vi "PH_SHS_Analysis_Calibrator.ProcState.vi"(0 "i ref in":refnum<vi>, 2 "state timeout":i32=-1, 4 "state":string, 5 "error in (no error)":errorcluster) -> (14 "i ref out":refnum<vi>, 18 "next state":string, 19 "error out":errorcluster)   [LabVIEW 2014, in "PH_SHS_Analysis_Calibrator.lvlib"]
doc: "This VI represents part of the internal state machine of the object. All methods that are needed to implement the required functionality of the state machine will be called from THIS VI. Add your code here."
uses:
  PH_SHS_Analysis_Calibrator.lvlib
  CSCore/CSSystem/CoreDefs/CoreDefs.error_type.ctl
  CSCore/CSSystem/CoreLib/CoreLib.lvlib
  CSCore/BaseSM/BaseSM.lvlib
  CSCore/BaseProcess/BaseProcess.lvlib
  CSCore/CSSystem/CSSystemLib/CSSystemLib.lvlib
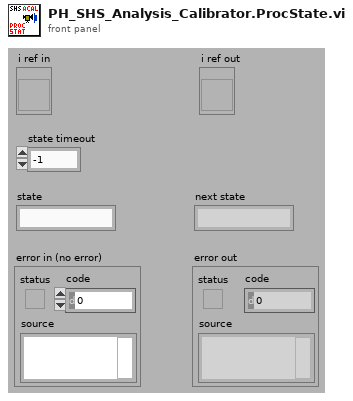
[diagram p1: front panel]
types:
  T1 = enum16{"simple", "synchronous", "asynchronous", "notification"}
  T2 = typedef "CoreDefs.error_type.ctl" = enum16{"no error", "can't load process", "can't unload process", "process does not exist", "can't install process", "can't remove process", "unknown function", "time out", "can't execute function", "duplicate queue name", "super not found", "caller queue invalid", "can't ping process", "unknown error", "VISA Error", "VISA timeout", "GPIB timeout", "GPIB error", "communication error", "data type mismatch", "can't read data from OPC server", "can't write data to OPC server", "OET error", "function not implemented", "process already exists", "invalid Shared Variable name", "error writing Shared Variable", "error reading Shared Variable", "invalid client name", "corrupt database", "unknown class", "call not authorized", "parameter out of range", "OET timeout: can't get data to modify", "invalid queue name", "requested operation incompatible with current state", "event undefined", "event disabled", "state undefined", "caller is not a friend", "EventBuilder: bad eventID", "EventBuilder: no DAQ devices", "a thread must not stop itself", "UNUSED ELEMENT4", "DiscArchiver: eventData incomplete", "DiscArchiver: eventData does not belong to run", "DiscArchiver: can't open file", "DiscArchiver: can't write to file", "DiscArchiver: available disc space low", "can't acquire semaphore", "error reading data from database", "notifier object is not existing", "can't register process", "can't unregister process", "illegal event type", "object disabled", "object already exists", "can't change state", "Instrument not found", "no connection to remote node", "invalid reference", "N/A", "UNUSED ELEMENT 1", "element not found", "illegal TCP/IP connection detected", "object does not exist", "invalid access ID", "unknown CS system", "invalid privilige", "unsupported data type", "unsupported server type", "IO server already exists", "Shared Variable already exists"}
  T3 = typedef "PH_SHS_Analysis_Calibrator.lvlib/PH_SHS_Analysis_Calibrator.i attribute.ctl" = cluster{"GUI Refs":cluster{"Available Cams":refnum<vi>, "OK":refnum<vi>, "Skip":refnum<vi>, "Repeat":refnum<vi>, "Cancel":refnum<vi>, "Dialog":refnum<vi>, "Enough Images?":refnum<vi>}, "Cam instances":string[], "Status":cluster{"#":i32, "Data calculated":bool, "Wanted #":i32}, "IMAQ Image Array":T4[], "Pixel Size [µm]":dbl, "MLA Pitch [µm]":dbl, "Method":enum16{"automatic", "manual"}, "Enough Images?":bool, "SHS Reference Result":T5, "Calculation Error":errorcluster}
  T4 = typedef "IMAQ Image.ctl" = refnum<image>
  T5 = typedef "SHS_Common.lvlib/SHSReference.ctl" = cluster{"Reference":T6[][], "Lens Array Pitch [px]":dbl}
  T6 = typedef "SHS_Common.lvlib/ReferencePoint.ctl" = cluster{"Rect":T7, "Point":T8}
  T7 = typedef "SHS_Common.lvlib/Rectangle.ctl" = cluster{"Left":i32, "Top":i32, "Right":i32, "Bottom":i32}
  T8 = typedef "SHS_Common.lvlib/Point.ctl" = cluster{"x":dbl, "y":dbl, "valid?":bool, "weight":dbl}
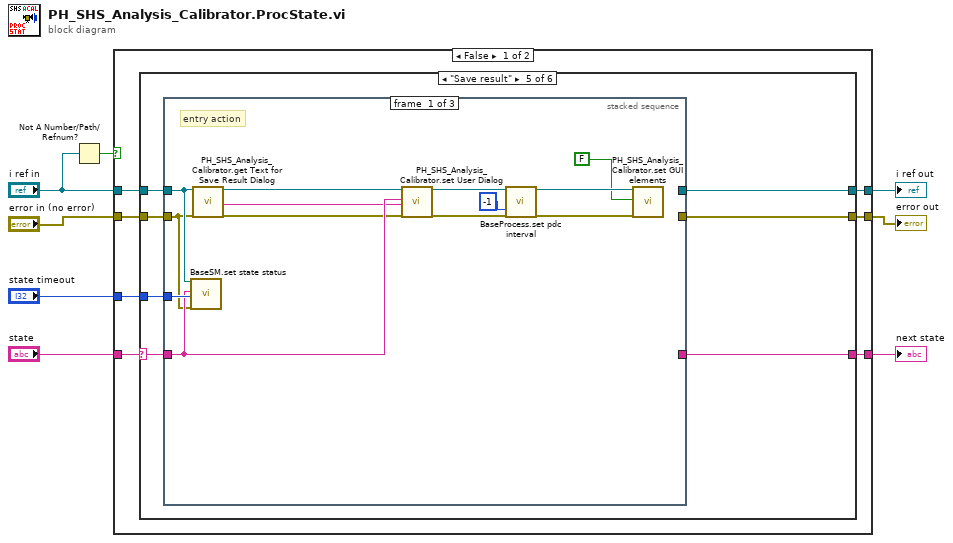
[diagram p0: block diagram]
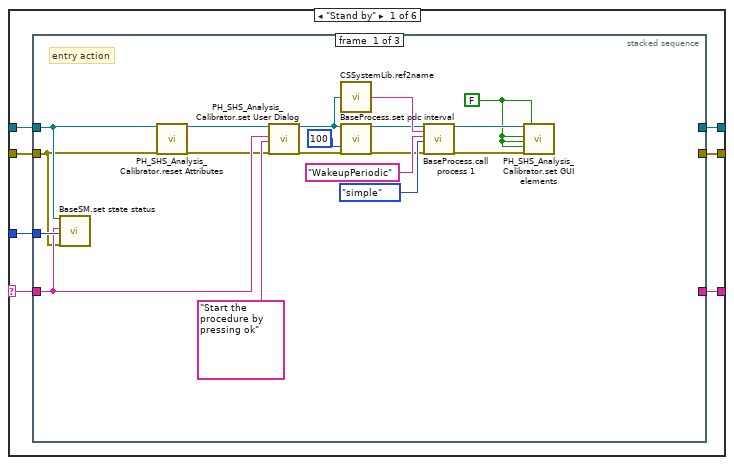
[diagram p2: hidden frame]
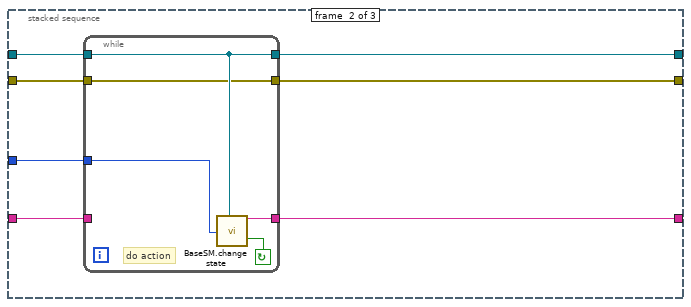
[diagram p3: hidden frame]
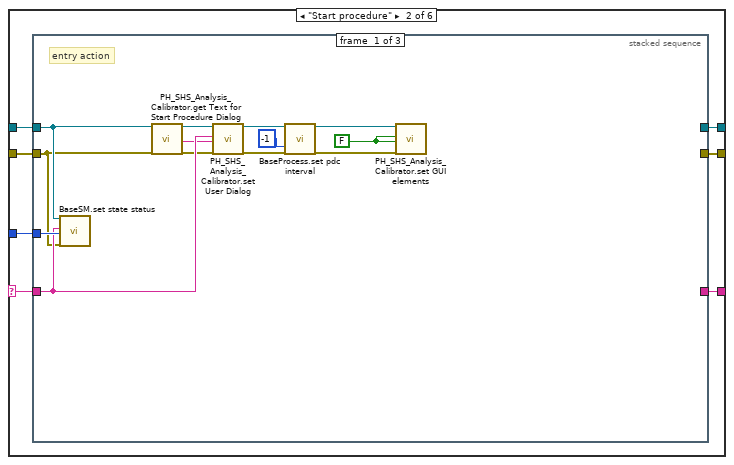
[diagram p5: hidden frame]
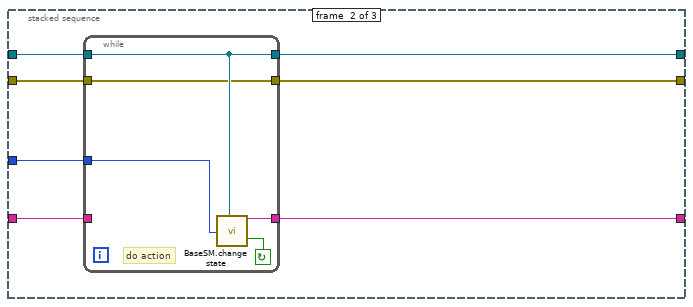
[diagram p6: hidden frame]
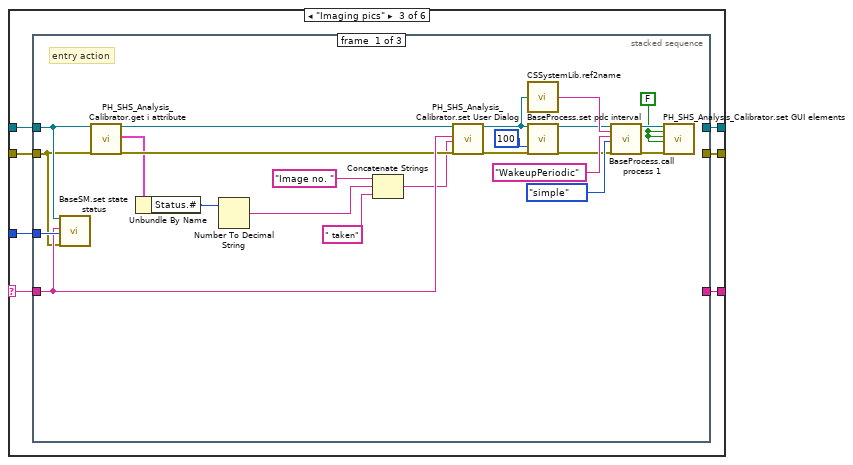
[diagram p8: hidden frame]
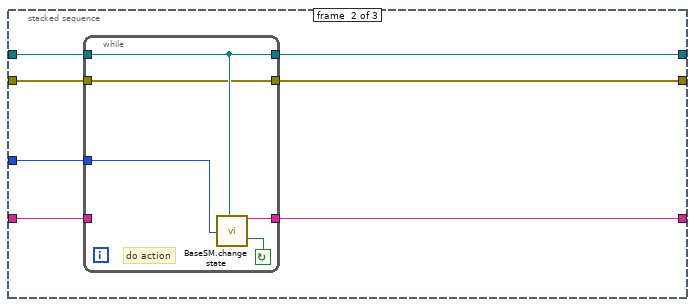
[diagram p9: hidden frame]
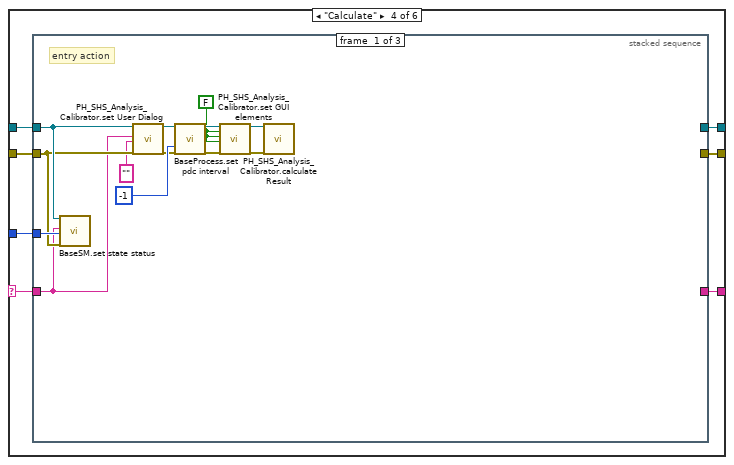
[diagram p11: hidden frame]
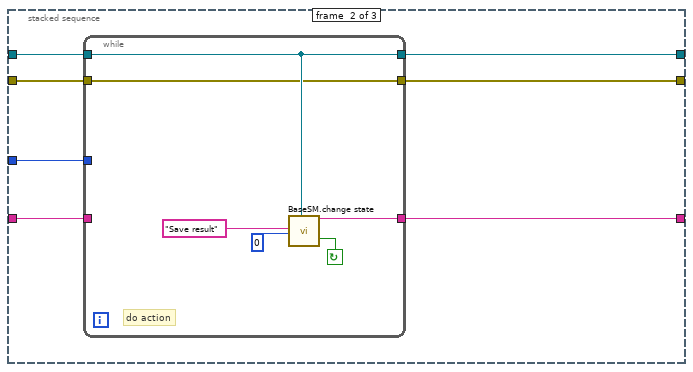
[diagram p12: hidden frame]
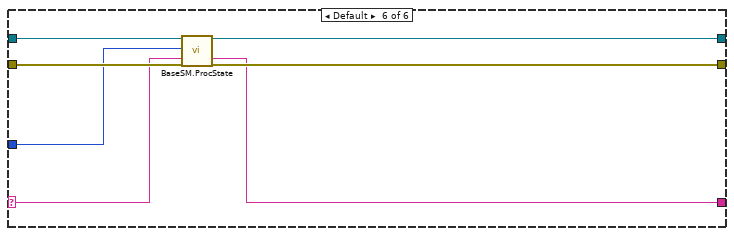
[diagram p16: hidden frame]
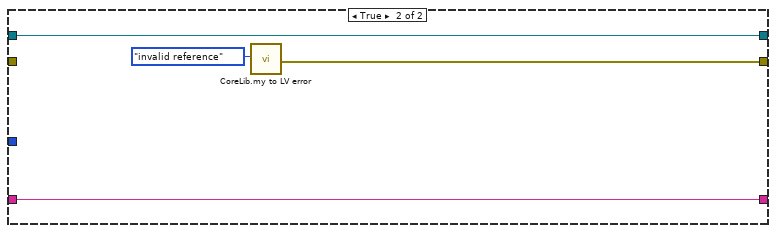
[diagram p17: hidden frame]
diagram:
  n1 = Not A Number/Path/Refnum?(number/path/refnum="i ref in") -> (NaN/Path/Refnum?=w2:bool)
  n2 = case shown="False" w2 {
    tunnel: "i ref in" -> [w15 w202]
    tunnel: [w14 w202] -> w8
    tunnel: "state" -> [w13 w199]
    tunnel: [w12 w199] -> w6
    tunnel: "state timeout" -> [w11 _]
    tunnel: "error in (no error)" -> [w10 _]
    tunnel: [w9 w200] -> w3
    frame False {
      n3 = case shown="\"Save result\"" w13 {
        selector: w13 -> [w22 w59 w91 w133 w166 w193]
        tunnel: w15 -> [w20 w57 w89 w131 w164 w198]
        tunnel: [w19 w56 w88 w130 w163 w197] -> w14
        tunnel: [w21 w58 w90 w132 w165 w192] -> w12
        tunnel: w11 -> [w18 w55 w87 w129 w162 w194]
        tunnel: w10 -> [w17 w54 w86 w128 w161 w196]
        tunnel: [w16 w53 w85 w127 w160 w195] -> w9
        frame "Stand by" {
          n4 = stacked-sequence {
            tunnel: w22 -> [w39 w47 _]
            tunnel: [_ w46 _] -> w21
            tunnel: w20 -> [w26 w44 _]
            tunnel: [_ w43 _] -> w19
            tunnel: w18 -> [w40 w45 _]
            tunnel: w17 -> [w24 w41 _]
            tunnel: [_ w42 _] -> w16
            frame #0 {
              w27 = FALSE ("Cams disabled (true)")
              # "entry action"
              n5 = call "BaseSM.set state status.vi"("i ref in"=w26, "stateStatus"=w39, "ms timeout (10000)"=w40, "error in (no error)"=w24) -> ()  [unwired: 13 in, 3 out]
              n6 = call "PH_SHS_Analysis_Calibrator.reset Attributes.vi"("i ref in"=w26, "error in (no error)"=w24) -> ("i ref out"=w25:refnum<vi>, "error out"=w23:errorcluster)  [unwired: 16 in]
              n7 = call "PH_SHS_Analysis_Calibrator.set User Dialog.vi"("i ref in"=w25, "State"=w39, "Text"="Start the procedure by pressing ok", "error in (no error)"=w23) -> ("i ref out"=w31:refnum<vi>, "error out"=w33:errorcluster)  [unwired: 14 in]
              n8 = call "CSSystemLib.ref2name.vi"("obj refnum"=w31) -> ("name"=w37:string)
              n9 = call "BaseProcess.set pdc interval.vi"("i ref in"=w31, "PeriodicInterval [ms]"=100 ("PeriodicInterval"), "error in (no error)"=w33) -> ("i ref out"=w32:refnum<vi>, "error out"=w34:errorcluster)  [unwired: 14 in, 1 out]
              n10 = call "BaseProcess.call process 1.vi"("i ref in"=w32, "Object"=w37, "Selector"="WakeupPeriodic", "CallType"=T1."simple", "error in (no error)"=w34) -> ("i ref out"=w29:refnum<vi>, "error out"=w28:errorcluster)  [unwired: 12 in, 1 out]
              n11 = call "PH_SHS_Analysis_Calibrator.set GUI elements.vi"("i ref in"=w29, "skip visible (true)"=w27, "Repeat visible (true)"=w27, "Cancel visible (true)"=w27, "error in (no error)"=w28, "Cams disabled (true)"=w27) -> ()  [unwired: 12 in, 2 out]
            }
            frame #1 {
              n12 = while {
                tunnel: w45 -> [w50]
                tunnel: [w52] -> w46
                tunnel: w47 -> [_]
                tunnel: w44 -> [w49]
                tunnel: [w49] -> w43
                tunnel: [w48] -> w42
                tunnel: w41 -> [w48]
                stop <- w51 continue-if-true
                # "do action"
                n13 = call "BaseSM.change state.vi"("wait time [ms]"=w50, "i ref in"=w49) -> ("next state"=w52:string, "continue loop"=w51:bool)  [unwired: 14 in, 2 out]
              }
            }
            frame #2 {
              # "exit action"
            }
          }
        }
        frame "Start procedure" {
          n14 = stacked-sequence {
            tunnel: w59 -> [w71 w79 _]
            tunnel: [_ w78 _] -> w58
            tunnel: w57 -> [w65 w76 _]
            tunnel: [_ w75 _] -> w56
            tunnel: w55 -> [w72 w77 _]
            tunnel: w54 -> [w63 w73 _]
            tunnel: [_ w74 _] -> w53
            frame #0 {
              w60 = FALSE ("Repeat visible (true)")
              # "entry action"
              n15 = call "BaseSM.set state status.vi"("i ref in"=w65, "stateStatus"=w71, "ms timeout (10000)"=w72, "error in (no error)"=w63) -> ()  [unwired: 13 in, 3 out]
              n16 = call "PH_SHS_Analysis_Calibrator.get Text for Start Procedure Dialog.vi"("i ref in"=w65, "error in (no error)"=w63) -> ("i ref out"=w64:refnum<vi>, "Dialog Start Procedure"=w61:string, "error out"=w62:errorcluster)  [unwired: 15 in]
              n17 = call "PH_SHS_Analysis_Calibrator.set User Dialog.vi"("i ref in"=w64, "State"=w71, "Text"=w61, "error in (no error)"=w62) -> ("i ref out"=w68:refnum<vi>, "error out"=w69:errorcluster)  [unwired: 14 in]
              n18 = call "BaseProcess.set pdc interval.vi"("i ref in"=w68, "PeriodicInterval [ms]"=-1 ("PeriodicInterval"), "error in (no error)"=w69) -> ("i ref out"=w67:refnum<vi>, "error out"=w66:errorcluster)  [unwired: 14 in, 1 out]
              n19 = call "PH_SHS_Analysis_Calibrator.set GUI elements.vi"("i ref in"=w67, "skip visible (true)"=w60, "Repeat visible (true)"=w60, "error in (no error)"=w66) -> ()  [unwired: 14 in, 2 out]
            }
            frame #1 {
              n20 = while {
                tunnel: w77 -> [w82]
                tunnel: [w84] -> w78
                tunnel: w79 -> [_]
                tunnel: w76 -> [w81]
                tunnel: [w81] -> w75
                tunnel: [w80] -> w74
                tunnel: w73 -> [w80]
                stop <- w83 continue-if-true
                # "do action"
                n21 = call "BaseSM.change state.vi"("wait time [ms]"=w82, "i ref in"=w81) -> ("next state"=w84:string, "continue loop"=w83:bool)  [unwired: 14 in, 2 out]
              }
            }
            frame #2 {
              # "exit action"
            }
          }
        }
        frame "Imaging pics" {
          n22 = stacked-sequence {
            tunnel: w91 -> [w113 w121 _]
            tunnel: [_ w120 _] -> w90
            tunnel: w89 -> [w112 w118 _]
            tunnel: [_ w117 _] -> w88
            tunnel: w87 -> [w114 w119 _]
            tunnel: w86 -> [w110 w115 _]
            tunnel: [_ w116 _] -> w85
            frame #0 {
              w92 = FALSE ("ok visible (true)")
              # "entry action"
              n23 = call "BaseSM.set state status.vi"("i ref in"=w112, "stateStatus"=w113, "ms timeout (10000)"=w114, "error in (no error)"=w110) -> ()  [unwired: 13 in, 3 out]
              n24 = call "PH_SHS_Analysis_Calibrator.get i attribute.vi"("i ref in"=w112, "error in (no error)"=w110) -> ("i ref out"=w111:refnum<vi>, "i attribute"=w108:T3, "error out"=w109:errorcluster)  [unwired: 15 in]
              n25 = Unbundle By Name(w108) -> ("Status.#"=w107:i32)
              n26 = Number To Decimal String(number=w107) -> (decimal integer string=w105:string)  [unwired: 1 in]
              n27 = Concatenate Strings("Image no. " ("string"), w105, " taken" ("string")) -> (w103:string)
              n28 = call "PH_SHS_Analysis_Calibrator.set User Dialog.vi"("i ref in"=w111, "State"=w113, "Text"=w103, "error in (no error)"=w109) -> ("i ref out"=w96:refnum<vi>, "error out"=w95:errorcluster)  [unwired: 14 in]
              n29 = call "CSSystemLib.ref2name.vi"("obj refnum"=w96) -> ("name"=w101:string)
              n30 = call "BaseProcess.set pdc interval.vi"("i ref in"=w96, "PeriodicInterval [ms]"=100 ("PeriodicInterval"), "error in (no error)"=w95) -> ("i ref out"=w97:refnum<vi>, "error out"=w98:errorcluster)  [unwired: 14 in, 1 out]
              n31 = call "BaseProcess.call process 1.vi"("i ref in"=w97, "Object"=w101, "Selector"="WakeupPeriodic", "CallType"=T1."simple", "error in (no error)"=w98) -> ("i ref out"=w94:refnum<vi>, "error out"=w93:errorcluster)  [unwired: 12 in, 1 out]
              n32 = call "PH_SHS_Analysis_Calibrator.set GUI elements.vi"("i ref in"=w94, "ok visible (true)"=w92, "skip visible (true)"=w92, "Repeat visible (true)"=w92, "error in (no error)"=w93) -> ()  [unwired: 13 in, 2 out]
            }
            frame #1 {
              n33 = while {
                tunnel: w119 -> [w124]
                tunnel: [w126] -> w120
                tunnel: w121 -> [_]
                tunnel: w118 -> [w123]
                tunnel: [w123] -> w117
                tunnel: [w122] -> w116
                tunnel: w115 -> [w122]
                stop <- w125 continue-if-true
                # "do action"
                n34 = call "BaseSM.change state.vi"("wait time [ms]"=w124, "i ref in"=w123) -> ("next state"=w126:string, "continue loop"=w125:bool)  [unwired: 14 in, 2 out]
              }
            }
            frame #2 {
              # "exit action"
            }
          }
        }
        frame "Calculate" {
          n35 = stacked-sequence {
            tunnel: w133 -> [w143 w153 _]
            tunnel: [_ w152 _] -> w132
            tunnel: w131 -> [w145 w150 _]
            tunnel: [_ w149 _] -> w130
            tunnel: w129 -> [w146 w151 _]
            tunnel: w128 -> [w144 w147 _]
            tunnel: [_ w148 _] -> w127
            frame #0 {
              w136 = FALSE ("ok visible (true)")
              # "entry action"
              n36 = call "BaseSM.set state status.vi"("i ref in"=w145, "stateStatus"=w143, "ms timeout (10000)"=w146, "error in (no error)"=w144) -> ()  [unwired: 13 in, 3 out]
              n37 = call "PH_SHS_Analysis_Calibrator.set User Dialog.vi"("i ref in"=w145, "State"=w143, "Text"="", "error in (no error)"=w144) -> ("i ref out"=w140:refnum<vi>, "error out"=w141:errorcluster)  [unwired: 14 in]
              n38 = call "BaseProcess.set pdc interval.vi"("i ref in"=w140, "PeriodicInterval [ms]"=-1 ("PeriodicInterval"), "error in (no error)"=w141) -> ("i ref out"=w139:refnum<vi>, "error out"=w138:errorcluster)  [unwired: 14 in, 1 out]
              n39 = call "PH_SHS_Analysis_Calibrator.set GUI elements.vi"("i ref in"=w139, "ok visible (true)"=w136, "skip visible (true)"=w136, "Repeat visible (true)"=w136, "error in (no error)"=w138) -> ("i ref out"=w135:refnum<vi>, "error out"=w134:errorcluster)  [unwired: 13 in]
              n40 = call "PH_SHS_Analysis_Calibrator.calculate Result.vi"("i ref in"=w135, "error in"=w134) -> ()  [unwired: 16 in, 2 out]
            }
            frame #1 {
              n41 = while {
                tunnel: w151 -> [_]
                tunnel: [w159] -> w152
                tunnel: w153 -> [_]
                tunnel: w150 -> [w157]
                tunnel: [w157] -> w149
                tunnel: [w156] -> w148
                tunnel: w147 -> [w156]
                stop <- w158 continue-if-true
                # "do action"
                n42 = call "BaseSM.change state.vi"("default state"="Save result", "wait time [ms]"=0, "i ref in"=w157) -> ("next state"=w159:string, "continue loop"=w158:bool)  [unwired: 13 in, 2 out]
              }
            }
            frame #2 {
              # "exit action"
            }
          }
        }
        frame "Save result" {
          n43 = stacked-sequence {
            tunnel: w166 -> [w178 w186 _]
            tunnel: [_ w185 _] -> w165
            tunnel: w164 -> [w170 w183 _]
            tunnel: [_ w182 _] -> w163
            tunnel: w162 -> [w179 w184 _]
            tunnel: w161 -> [w168 w180 _]
            tunnel: [_ w181 _] -> w160
            frame #0 {
              # "entry action"
              n44 = call "BaseSM.set state status.vi"("i ref in"=w170, "stateStatus"=w178, "ms timeout (10000)"=w179, "error in (no error)"=w168) -> ()  [unwired: 13 in, 3 out]
              n45 = call "PH_SHS_Analysis_Calibrator.get Text for Save Result Dialog.vi"("i ref in"=w170, "error in (no error)"=w168) -> ("i ref out"=w169:refnum<vi>, "User Dialog"=w172:string, "error out"=w167:errorcluster)  [unwired: 15 in]
              n46 = call "PH_SHS_Analysis_Calibrator.set User Dialog.vi"("i ref in"=w169, "State"=w178, "Text"=w172, "error in (no error)"=w167) -> ("i ref out"=w175:refnum<vi>, "error out"=w176:errorcluster)  [unwired: 14 in]
              n47 = call "BaseProcess.set pdc interval.vi"("i ref in"=w175, "PeriodicInterval [ms]"=-1 ("PeriodicInterval"), "error in (no error)"=w176) -> ("i ref out"=w174:refnum<vi>, "error out"=w173:errorcluster)  [unwired: 14 in, 1 out]
              n48 = call "PH_SHS_Analysis_Calibrator.set GUI elements.vi"("i ref in"=w174, "skip visible (true)"=FALSE, "error in (no error)"=w173) -> ()  [unwired: 15 in, 2 out]
            }
            frame #1 {
              n49 = while {
                tunnel: w184 -> [w187]
                tunnel: [w191] -> w185
                tunnel: w186 -> [_]
                tunnel: w183 -> [w189]
                tunnel: [w189] -> w182
                tunnel: [w188] -> w181
                tunnel: w180 -> [w188]
                stop <- w190 continue-if-true
                # "do action"
                n50 = call "BaseSM.change state.vi"("wait time [ms]"=w187, "i ref in"=w189) -> ("next state"=w191:string, "continue loop"=w190:bool)  [unwired: 14 in, 2 out]
              }
            }
            frame #2 {
              # "exit action"
            }
          }
        }
        frame Default {
          n51 = call "BaseSM.ProcState.vi"("i ref in"=w198, "state timeout [ms]"=w194, "state"=w193, "error in (no error)"=w196) -> ("i ref out"=w197:refnum<vi>, "next state"=w192:string, "error out"=w195:errorcluster)  [unwired: 13 in]
        }
      }
    }
    frame True {
      n52 = call "CoreLib.my to LV error.vi"("ErrorTypes"=CoreDefs.error_type."invalid reference") -> ("myErrorCluster"=w200:errorcluster)  [unwired: 17 in, 1 out]
    }
  }
  "i ref out" <- w8
  "next state" <- w6
  "error out" <- w3
